vi "CellValidating Event Callback.vi"(4 "DataGridView in":refnum<class "DataGridView.lvclass">, 5 "Event Data":cluster{"sender":refnum<k24>, "e":refnum<k24>}, 6 "Control Ref":refnum<k24>, 7 "Event Common Data":T1) -> ()   [LabVIEW 2013, in "DataGrid.lvlib" / "DataGridView.lvclass"]
uses:
  DataGridView/DataGridView.lvclass
  System.Windows.Forms
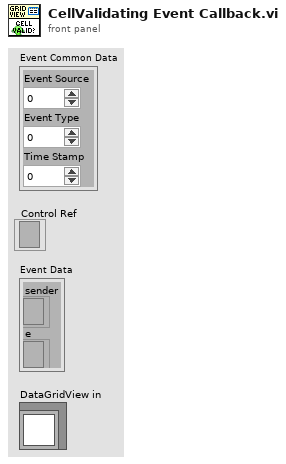
[diagram p1: front panel]
types:
  T1 = cluster{"Event Source":i32, "Event Type":u32, "Time Stamp":u32}
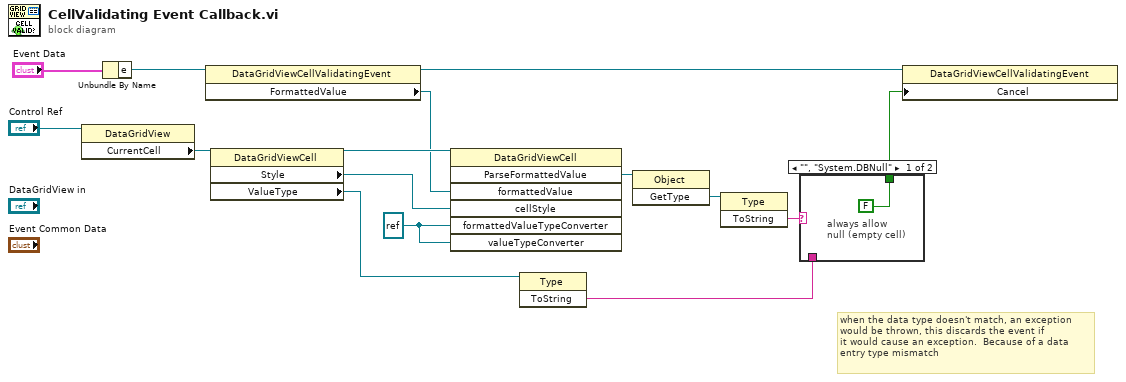
[diagram p0: block diagram]
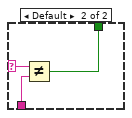
[diagram p2: hidden frame]
diagram:
  w6 = refnum<k24> refnum ("formattedValueTypeConverter")
  # "when the data type doesn't match, an exception\nwould be thrown, this discards the event if\nit would cause an exception.  Because of a data \nentry type mismatch"
  n1 = property class="DataGridView"(reference="Control Ref") -> ("CurrentCell"=w14:refnum<k24>)  [unwired: 1 in, 2 out]
  n2 = Unbundle By Name("Event Data") -> ("e"=w12:refnum<k24>)
  n3 = property class="DataGridViewCellValidatingEvent"(reference=w12) -> (reference out=w10:refnum<k24>, "FormattedValue"=w8:refnum<k24>)  [unwired: 1 in, 1 out]
  n4 = property class="DataGridViewCell"(reference=w14) -> (reference out=w9:refnum<k24>, "Style"=w4:refnum<k24>, "ValueType"=w5:refnum<k24>)  [unwired: 1 in, 1 out]
  n5 = invoke class="DataGridViewCell" method="ParseFormattedValue"(reference=w9, "formattedValue"=w8, "cellStyle"=w4, "formattedValueTypeConverter"=w6, "valueTypeConverter"=w6) -> ("ParseFormattedValue"=w7:refnum<k24>)  [unwired: 2 in, 6 out]
  n6 = invoke class="Type" method="ToString"(reference=w5) -> ("ToString"=w1:string)  [unwired: 2 in, 2 out]
  n7 = invoke class="Object" method="GetType"(reference=w7) -> ("GetType"=w11:refnum<k24>)  [unwired: 2 in, 2 out]
  n8 = invoke class="Type" method="ToString"(reference=w11) -> ("ToString"=w2:string)  [unwired: 2 in, 2 out]
  n9 = case shown="\"\", \"System.DBNull\"" w2 {
    selector: w2 -> [_ w18]
    tunnel: w1 -> [_ w19]
    tunnel: [FALSE w17] -> w3
    frame "", "System.DBNull" {
      # "always allow\nnull (empty cell)"
    }
    frame Default {
      n10 = Not Equal?(x=w18, y=w19) -> (x != y?=w17:bool)
    }
  }
  n11 = property class="DataGridViewCellValidatingEvent"(reference=w10, "Cancel"=w3) -> ()  [unwired: 1 in, 2 out]
